vi "GenerateValveSequenceMultiMix.vi"(6 "Mix Water Valve":u16(ring)=12 items=["A1", "A2", "A3", "A4", "B1", "B2", "B3", "B4", "B5", "B6", "B7", "B8", "A5", "A6", "A7", "A8"], 8 "Ctr Water Valve":u16(ring)=15 items=["A1", "A2", "A3", "A4", "B1", "B2", "B3", "B4", "B5", "B6", "B7", "B8", "A5", "A6", "A7", "A8"], 9 "Ctr Odor Valve":u16(ring)=14 items=["A1", "A2", "A3", "A4", "B1", "B2", "B3", "B4", "B5", "B6", "B7", "B8", "A5", "A6", "A7", "A8"], 10 "Valves":u16[](array[ring])=[0, 1, 2, 3, 8, 9, 10, 11, 4, 5, 6, 7, 8] items=["A1", "A2", "A3", "A4", "B1", "B2", "B3", "B4", "B5", "B6", "B7", "B8"], 11 "Mix Sequence Array":bool[][](array[boolean])) -> (3 "Valve Sequence Data":T1(array[cluster]))   [LabVIEW 2016]
uses:
  <vilib>/imath/engines/lvmath2/RunTimeEngine/VariableToken/Support/NIMS_Vector Boolean Index to I32 Index.vi
  <vilib>/imath/engines/lvmath2/RunTimeEngine/IndexRead/NIMS V(V).vi
  <instcachedir>/0/NIMS V(V)_298D9CB7BFEB42B8BC8D9C3C28AE8C70.lvgen/NIMS V(V)_298D9CB7BFEB42B8BC8D9C3C28AE8C70_001.vi
  <vilib>/imathl/engines/lvmath/Functions/Error Handling/Create Error.vi
  <vilib>/imath/engines/lvmath2/RunTimeEngine/NodeEndStatement/NIMS_NodeEndStatement_Output.vi
  <instcachedir>/0/NIMS_NodeEndStatement_Output_53EC0D466D134D7ABD903AC30B43404B.lvgen/NIMS_NodeEndStatement_Output_53EC0D466D134D7ABD903AC30B43404B_011.vi
  <vilib>/imath/engines/lvmath2/RunTimeEngine/ErrorHandling/NIMS_Finalize Error.vi
panel:
  in  "Max Number of\nOdors in Mixture":u16=10
  out "Array":cluster{u16[]}[](array[cluster])
  in  "Flowboard":enum16{"A", "B", "C"}(ring)
  in  "Channel":enum16{"1", "2", "3", "4", "5", "6", "7", "8"}(ring)
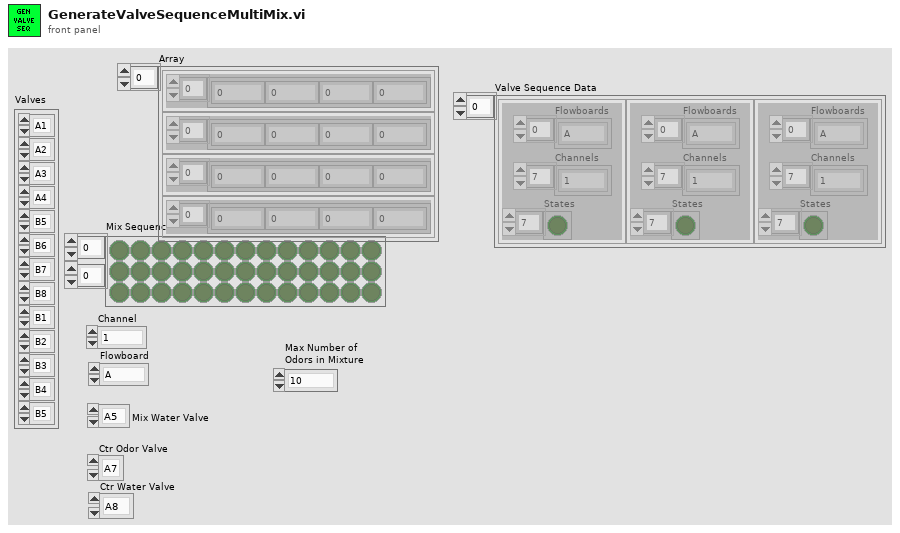
[diagram p1: front panel]
types:
  T1 = cluster{"Flowboards":enum16{"A", "B", "C"}[], "Channels":enum16{"1", "2", "3", "4", "5", "6", "7", "8"}[], "States":bool[]}[]
  T2 = cluster{"Flowboards":enum16{"A", "B", "C"}[], "Channels":enum16{"1", "2", "3", "4", "5", "6", "7", "8"}[], "States":bool[]}
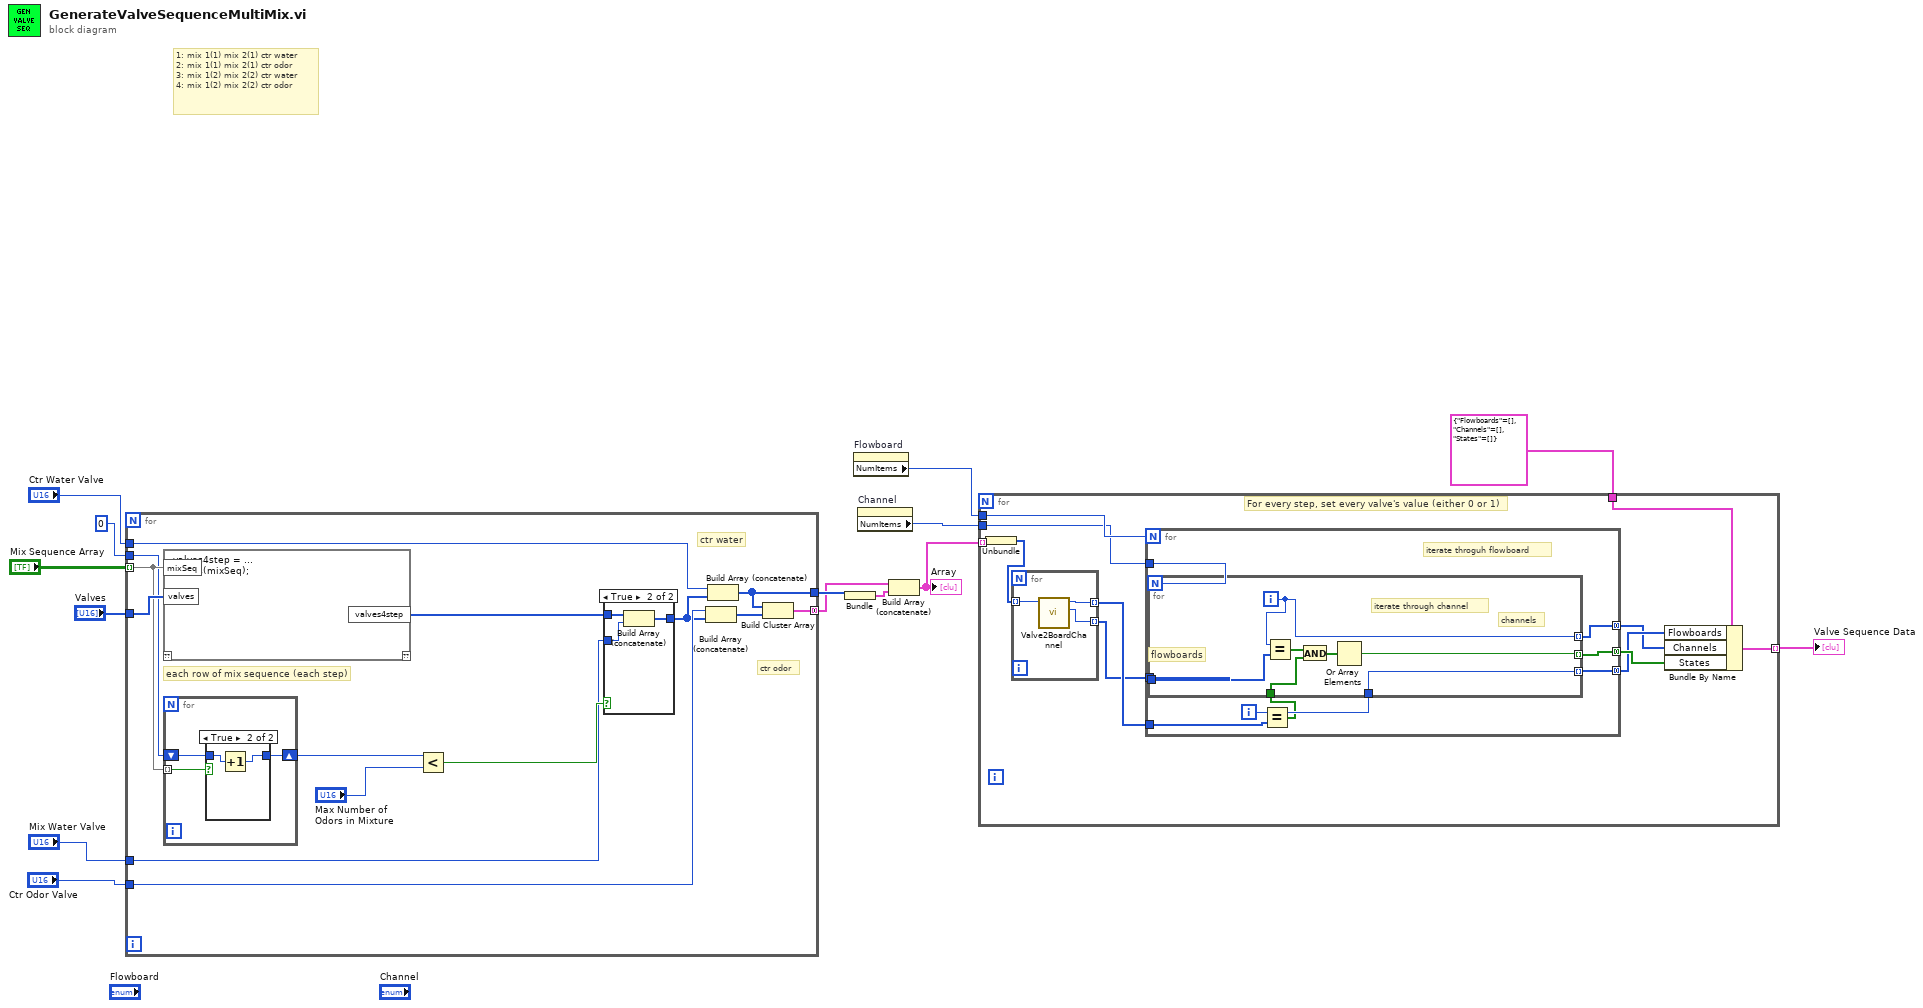
[diagram p0: block diagram]
diagram:
  # "1: mix 1(1) mix 2(1) ctr water\n2: mix 1(1) mix 2(1) ctr odor\n3: mix 1(2) mix 2(2) ctr water\n4: mix 1(2) mix 2(2) ctr odor"
  n1 = for {
    tunnel: "Mix Sequence Array" -> [w22] mode=indexing
    tunnel: "Valves" -> [w28]
    tunnel: "Ctr Water Valve" -> [w27]
    tunnel: "Ctr Odor Valve" -> [w26]
    tunnel: [w24] -> w5 mode=concatenating
    tunnel: [w23] -> w7
    tunnel: 0 -> [w21]
    tunnel: "Mix Water Valve" -> [w16]
    # "ctr odor"
    # "ctr water"
    # "each row of mix sequence (each step)"
    n2 = mathscript code="valves4step = ...\nvalves(mixSeq);"("mixSeq"=w22, "valves"=w28) -> ("valves4step"=w17:u16[])  [unwired: 1 in, 1 out]
    n3 = for {
      tunnel: w22 -> [w35] mode=indexing
      shift-right: [w33] -> w20
      shift-left: w21 -> [w34]
      n4 = case shown="True" w35 {
        tunnel: w34 -> [w36 w38]
        tunnel: [w36 w37] -> w33
        frame False {
        }
        frame True {
          n5 = Increment(x=w38) -> (x+1=w37:i32)
        }
      }
    }
    n6 = Less?(x=w20, y="Max Number of\nOdors in Mixture") -> (x < y?=w18:bool)
    n7 = case shown="True" w18 {
      tunnel: w17 -> [w29 w32]
      tunnel: w16 -> [_ w31]
      tunnel: [w29 w30] -> w15
      frame False {
      }
      frame True {
        n8 = Build Array (concatenate)(w32, w31) -> (w30:u16[])
      }
    }
    n9 = Build Array (concatenate)(w26, w15) -> (w25:u16[])
    n10 = Build Array (concatenate)(w27, w15) -> (w23:u16[])
    n11 = Build Cluster Array(w23, w25) -> (w24:cluster{u16[]}[])
  }
  n12 = Bundle(w7) -> (w6:cluster{u16[]})  [unwired: 1 in]
  n13 = property on="Flowboard" class="Enum (strict)"() -> ("NumItems"=w14:u32)  [unwired: 2 in, 2 out]
  n14 = property on="Channel" class="Enum (strict)"() -> ("NumItems"=w13:u32)  [unwired: 2 in, 2 out]
  n15 = Build Array (concatenate)(w5, w6) -> (w4:cluster{u16[]}[])
  "Array" <- w4
  n16 = for {
    tunnel: w14 -> [w82]
    tunnel: w13 -> [w81]
    tunnel: T2 {"Flowboards"=[], "Channels"=[], "States"=[]} ("Valve Data") -> [w80]
    tunnel: [w76] -> w3 mode=indexing
    tunnel: w4 -> [w75] mode=indexing
    # "For every step, set every valve's value (either 0 or 1)"
    n17 = Unbundle(w75) -> (w74:u16[])
    n18 = for {
      tunnel: [w85] -> w73 mode=indexing
      tunnel: w74 -> [w84] mode=indexing
      tunnel: [w83] -> w72 mode=indexing
      n19 = call "Valve2BoardChannel.vi"("ValveID"=w84) -> ("Channel"=w83:enum16{"1", "2", "3", "4", "5", "6", "7", "8"}, "Flowboard"=w85:enum16{"A", "B", "C"})  [unwired: 9 in]
    }
    n20 = for {
      N: w82 -> [_]
      tunnel: w81 -> [w93]
      tunnel: [w92] -> w77 mode=concatenating
      tunnel: [w91] -> w78 mode=concatenating
      tunnel: w73 -> [w89]
      tunnel: w72 -> [w90]
      tunnel: [w86] -> w79 mode=concatenating
      i -> [w88]
      # "iterate throguh flowboard"
      n21 = Equal?(x=w88, y=w89) -> (x = y?=w87:bool[])
      n22 = for {
        N: w93 -> [_]
        tunnel: [w99] -> w92 mode=indexing
        tunnel: w88 -> [w98]
        tunnel: [w98] -> w91 mode=indexing
        tunnel: w90 -> [w100]
        tunnel: w87 -> [w96]
        tunnel: [w94] -> w86 mode=indexing
        i -> [w99]
        # "flowboards"
        # "channels"
        # "iterate through channel"
        n23 = Equal?(x=w99, y=w100) -> (x = y?=w97:bool[])
        n24 = And(x=w97, y=w96) -> (x .and. y?=w95:bool[])
        n25 = Or Array Elements(Boolean array=w95) -> (logical OR=w94:bool)
      }
    }
    n26 = Bundle By Name(cluster=w80, "Flowboards"=w78, "Channels"=w77, "States"=w79) -> (w76:T2)
  }
  "Valve Sequence Data" <- w3
